vi "UnitTest-Logic.vi"(8 "error in (no error)":errorcluster, 9 "LV Data":T1={"Numeric Data"=100, "Float Data"=100.123, "String Data"="This is string", "Enum Data"=enum."Enum Item 2", "Array Data"=[1234, 2345, 3456, 4567]}, 10 "TableLogger Config":T2={"TableLogger"=enum."CSV Logger", "DB File Path"=path "C:/LogAnyLVdata/Test.csv", "DB Backup Config"={"Directory"=path "C:/LogAnyLVdata/dBbackup", "UTC Time Format"=FALSE, "On Launch"=FALSE, "Interval (Hours)"=0.01, "Size Multiples (Bytes)"=10000}}) -> (0 "error out":errorcluster, 3 "Test Result":bool)   [LabVIEW 2014]
uses:
  TableLogger_Actor/TableLoggerConfig.ctl
  TableLogger_Actor/TableLoggerTypes.ctl
  TableLogger_Actor/TableLoggerBackupConfig.ctl
  TableLogger_Actor/TableLoggerDataCluster.ctl
  TableLogger_Actor/Messages/InsertData_Msg/InsertData Msg.lvclass/InsertData Msg.ctl
  <vilib>/ActorFramework/Message Enqueuer/Message Enqueuer.lvclass/Message Enqueuer.ctl
  <vilib>/ActorFramework/Message Enqueuer/Enqueue.vi
  <vilib>/ActorFramework/Message Priority Queue/Priority Enqueue.vi
  TableLogger_Actor/Messages/InsertData_Msg/InsertData Msg.lvclass
  <vilib>/ActorFramework/Stop Msg/Stop Msg.lvclass
  TableLogger_Actor/TableLogger_Actor/TableLogger_Actor.lvclass
  TableLogger_Actor/TableLogger_Actor.lvlib
panel:
  # "Connector Pane"
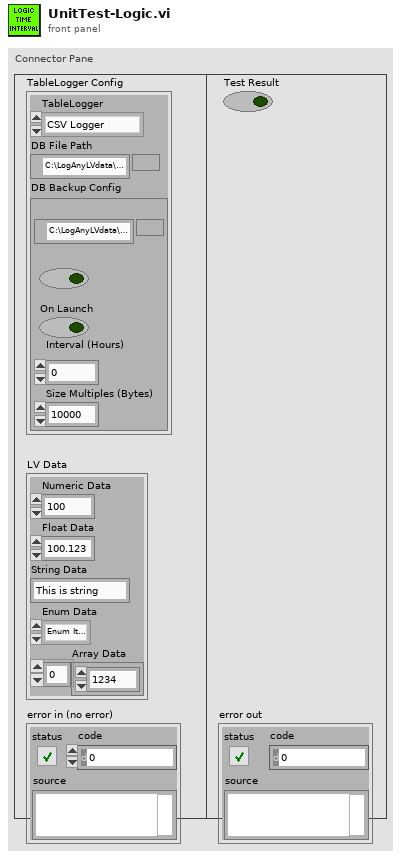
[diagram p1: front panel]
types:
  T1 = typedef "TableLogger_Actor.lvlib/TableLoggerDataCluster.ctl" = cluster{"Numeric Data":i32, "Float Data":dbl, "String Data":string, "Enum Data":enum16{"Enum Item 1", "Enum Item 2"}, "Array Data":i32[]}
  T2 = typedef "TableLogger_Actor.lvlib/TableLoggerConfig.ctl" = cluster{"TableLogger":T3, "DB File Path":path, "DB Backup Config":T4}
  T3 = typedef "TableLogger_Actor.lvlib/TableLoggerTypes.ctl" = enum16{"CSV Logger", "SQLite Logger"}
  T4 = typedef "TableLogger_Actor.lvlib/TableLoggerBackupConfig.ctl" = cluster{"Directory":path, "UTC Time Format":bool, "On Launch":bool, "Interval (Hours)":dbl, "Size Multiples (Bytes)":i32}
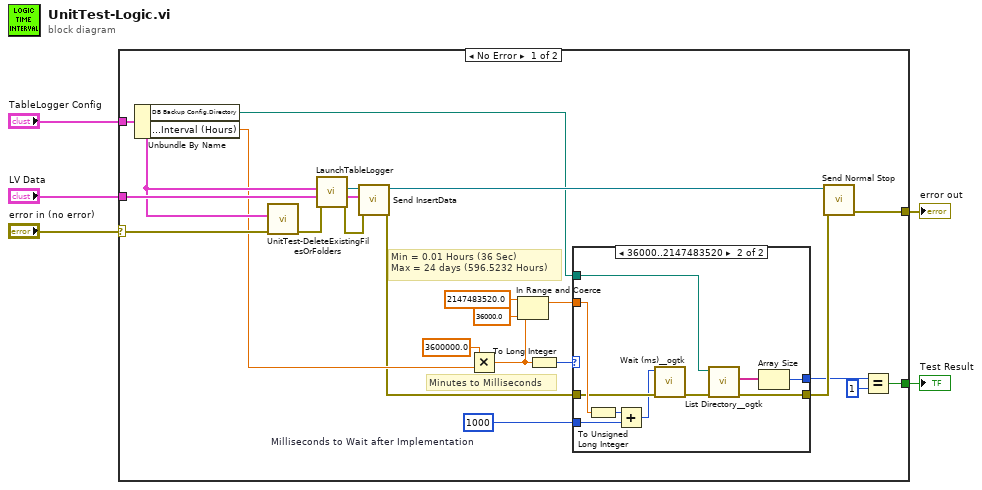
[diagram p0: block diagram]
diagram:
  n1 = case shown="No Error" "error in (no error)" {
    selector: "error in (no error)" -> [w24 w39]
    tunnel: [w27 _] -> w5
    tunnel: "LV Data" -> [w26 _]
    tunnel: "TableLogger Config" -> [w18 _]
    tunnel: [w23 w39] -> w1
    frame No Error {
      w9 = u32 1000  # Milliseconds to Wait after Implementation
      # "Min = 0.01 Hours (36 Sec)\nMax = 24 days (596.5232 Hours)"
      # "Minutes to Milliseconds"
      n2 = Unbundle By Name(w18) -> ("DB Backup Config.Directory"=w8:path, "DB Backup Config.Interval (Hours)"=w11:dbl)
      n3 = call "UnitTest-DeleteExistingFilesOrFolders.vi"("error in (no error)"=w24, "Config IN"=w18) -> ("error out"=w21:errorcluster)  [unwired: 9 in]
      n4 = call "LaunchTableLogger.vi"("error in (no error)"=w21, "Data Cluster (for Headers)"=w26, "TableLogger Config"=w18) -> ("error out"=w19:errorcluster, "TableLogger Actor's Enqueuer"=w20:refnum<class "Message Enqueuer.lvclass">)  [unwired: 5 in, 2 out]
      n5 = call "Send InsertData.vi"("error in (no error)"=w19, "Data"=w26, "Message Enqueuer"=w20) -> ("error out"=w10:errorcluster, "Message Enqueuer out"=w22:refnum<class "Message Enqueuer.lvclass">)  [unwired: 7 in]
      n6 = Multiply(x=3600000.0, y=w11) -> (x*y=w17:dbl)
      n7 = In Range and Coerce(upper limit=2147483520.0, x=w17, lower limit=36000.0) -> (coerced(x)=w16:dbl)  [unwired: 1 out]
      n8 = To Long Integer(number=w17) -> (32bit integer=w13:i32)
      n9 = case shown="36000..2147483520" w13 {
        tunnel: w10 -> [w28 w31]
        tunnel: [w28 w32] -> w7
        tunnel: w16 -> [_ w37]
        tunnel: w9 -> [_ w36]
        tunnel: w8 -> [_ w33]
        tunnel: [_ w29] -> w6
        frame ..0, Default {
        }
        frame 36000..2147483520 {
          n10 = To Unsigned Long Integer(number=w37) -> (unsigned 32bit integer=w38:u32)
          n11 = Add(x=w38, y=w36) -> (x+y=w30:u32)
          n12 = call <userlib>:"Wait (ms)__ogtk.vi"("error in (no error)"=w31, "milliseconds to wait"=w30) -> ("error out"=w34:errorcluster)  [unwired: 8 in, 1 out]
          n13 = call <userlib>:"List Directory__ogtk.vi"("error in (no error)"=w34, "directory path"=w33) -> ("error out"=w32:errorcluster, "file names"=w35:string[])  [unwired: 2 in, 2 out]
          n14 = Array Size(array=w35) -> (size(s)=w29:i32)
        }
      }
      n15 = call <vilib>:"Send Normal Stop.vi"("error in (no error)"=w7, "Message Enqueuer"=w22) -> ("error out"=w23:errorcluster)  [unwired: 9 in]
      n16 = Equal?(x=w6, y=1 ("x")) -> (x = y?=w27:bool)
    }
    frame Error {
    }
  }
  "Test Result" <- w5
  "error out" <- w1
